vi "Send speed logging notifier cases.vi"(8 "error in":errorcluster, 9 "Log speed data = T (Unused)":bool=TRUE, 11 "Logging queue element":T1={"Imaging Protocol"=enum."Live Imaging", "Number of Trials"=0, "Frame Size"=512, "# Averaged frames"=0, "Dwell time (us)"=0.0, "Index of Z-plane"=0, "Timelapse?"=FALSE, "Logging process is active"=FALSE, "Speed logging enabled"=FALSE, "tdms file ref"=refnum, "path"=path "", "Trial Number"=0, "Expected # points acquired"=FALSE, "Manually stopped"=FALSE, "Last trial"=FALSE, "Ch0 data"=[], "Ch1 data"=[], "Image Time"=[], "Continuous Time"=[], "Points acquired"={"Ch0 last trial"=0, "Ch1 last trial"=0, "All trials"=0}, "HW Timings File"=refnum} {"Frame Size" items=["100X100"=100, "128X128"=128, "200X200"=200, "256X256"=256, "512X512"=512, "1024x1024"=1024, "2048x2048"=2048]; "Dwell time (us)" format="%#.6g"}) -> (0 "error out":errorcluster)   [LabVIEW 2017]
uses:
  Typedefs/Logging queue element.ctl
  Typedefs/Imaging Protocols enum.ctl
  Typedefs/Frame Size.ctl
  Typedefs/Acquired points count.ctl
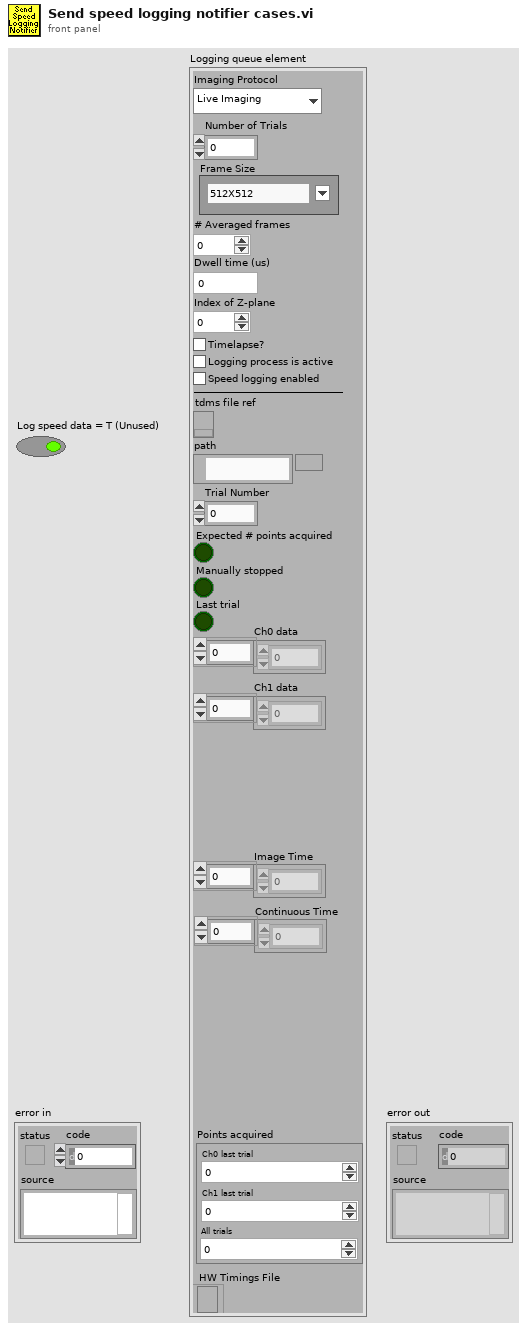
[diagram p1: front panel]
types:
  T1 = typedef "Logging queue element.ctl" = cluster{"Imaging Protocol":T2, "Number of Trials":u16, "Frame Size":T3, "# Averaged frames":u16, "Dwell time (us)":dbl, "Index of Z-plane":i32, "Timelapse?":bool, "Logging process is active":bool, "Speed logging enabled":bool, "tdms file ref":refnum<k34>, "path":path, "Trial Number":i32, "Expected # points acquired":bool, "Manually stopped":bool, "Last trial":bool, "Ch0 data":u32[], "Ch1 data":u32[], "Image Time":u64[], "Continuous Time":u64[], "Points acquired":T4, "HW Timings File":refnum<file>}
  T2 = typedef "Imaging Protocols enum.ctl" = enum16{"AOL Z-Stack", "Motor Z Stack", "Functional Acquisition", "Single Plane Acquisition", "Volume Acquisition", "Live Imaging", "Live Plane Imaging", "Live Volume Imaging"}
  T3 = typedef "Frame Size.ctl" = u16
  T4 = typedef "Acquired points count.ctl" = cluster{"Ch0 last trial":u64, "Ch1 last trial":u64, "All trials":u64}
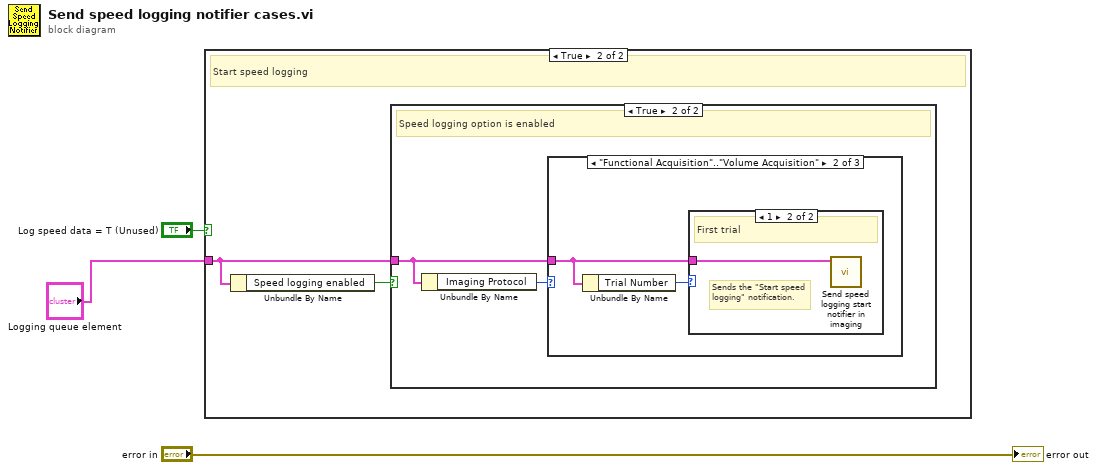
[diagram p0: block diagram]
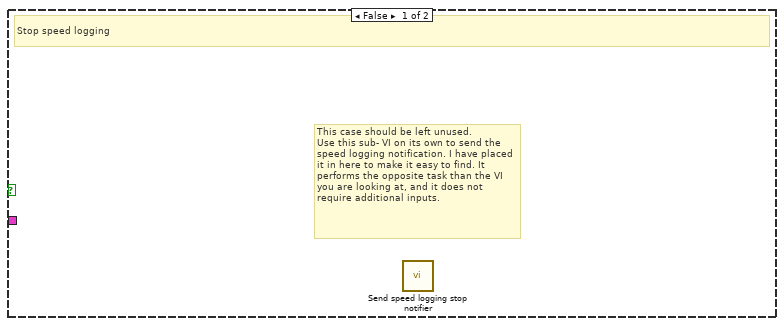
[diagram p2: hidden frame]
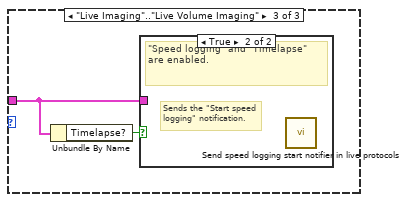
[diagram p6: hidden frame]
diagram:
  n1 = case shown="True" "Log speed data = T (Unused)" {
    tunnel: "Logging queue element" -> [_ w5]
    frame False {
      # "This case should be left unused.\nUse this sub- VI on its own to send the speed logging notification. I have placed it in here to make it easy to find. It performs the opposite task than the VI you are looking at, and it does not require additional inputs."
      # "Stop speed logging"
      n2 = call "Send speed logging stop notifier.vi"() -> ()  [unwired: 11 in, 1 out]
    }
    frame True {
      # "Start speed logging"
      n3 = Unbundle By Name(w5) -> ("Speed logging enabled"=w4:bool)
      n4 = case shown="True" w4 {
        tunnel: w5 -> [_ w6]
        frame False {
          # "Speed logging option is disabled"
        }
        frame True {
          # "Speed logging option is enabled"
          n5 = Unbundle By Name(w6) -> ("Imaging Protocol"=w7:T2)
          n6 = case shown="\"Functional Acquisition\"..\"Volume Acquisition\"" w7 {
            tunnel: w6 -> [_ w9 w12]
            frame Default {
            }
            frame "Functional Acquisition".."Volume Acquisition" {
              n7 = Unbundle By Name(w9) -> ("Trial Number"=w8:i32)
              n8 = case shown="1" w8 {
                tunnel: w9 -> [_ w10]
                frame Default {
                  # "Not the first trial"
                }
                frame 1 {
                  # "Sends the \"Start speed logging\" notification."
                  # "First trial"
                  n9 = call "Send speed logging start notifier in imaging.vi"("Logging queue element"=w10) -> ()  [unwired: 11 in]
                }
              }
            }
            frame "Live Imaging".."Live Volume Imaging" {
              n10 = Unbundle By Name(w12) -> ("Timelapse?"=w11:bool)
              n11 = case shown="True" w11 {
                tunnel: w12 -> [_ _]
                frame False {
                  # "\"Speed logging\" or \"Timelapse\" is disabled."
                }
                frame True {
                  # "Sends the \"Start speed logging\" notification."
                  # "\"Speed logging\" and \"Timelapse\" are enabled."
                  n12 = call "Send speed logging start notifier in live protocols.vi"() -> ()  [unwired: 12 in]
                }
              }
            }
          }
        }
      }
    }
  }
  "error out" <- "error in"
